vi "Get Variables.vi"(8 "error in (no error)":errorcluster, 11 "Booelan Operations in":refnum<class "Boolean Operations.lvclass">) -> (0 "error out":errorcluster, 2 "Variables":variant, 3 "Booelan Operations out":refnum<class "Boolean Operations.lvclass">)   [LabVIEW 2016, in "Boolean Operations.lvclass"]
uses:
  Boolean Operations.lvclass
  Boolean Operations.lvclass/Boolean Operations.ctl
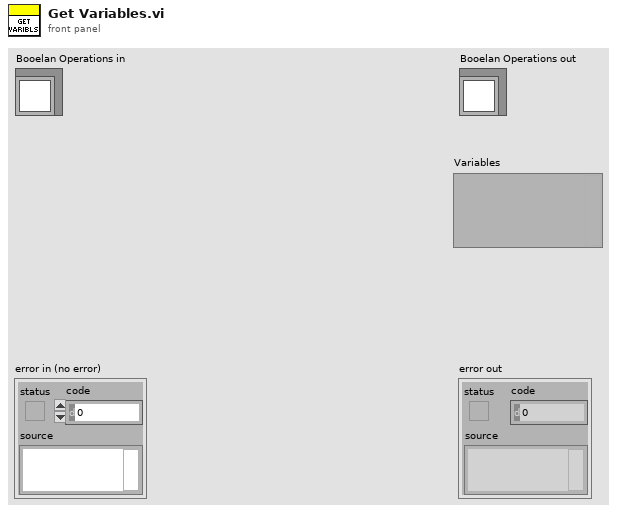
[diagram p1: front panel]
types:
  T1 = typedef "Boolean Operations.lvclass/Variables.ctl" = cluster{"Var1":bool, "Var2":bool}
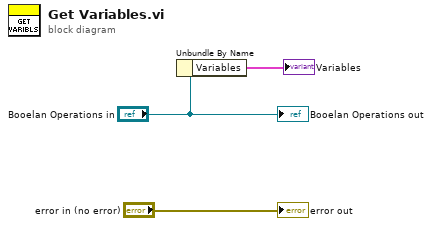
[diagram p0: block diagram]
diagram:
  n1 = Unbundle By Name("Booelan Operations in") -> ("Variables"=→"Variables":T1)
  "error out" <- "error in (no error)"
  "Booelan Operations out" <- "Booelan Operations in"
